vi "系统设置.vi"() -> ()   [LabVIEW 2016]
uses:
  <vilib>/Utility/miscctls.llb/LVPointTypeDef.ctl
  <vilib>/ptbypt/NI_PtbyPt.lvlib
  <vilib>/Utility/config.llb/NI_LVConfig.lvlib
  PLC/PLC.lvlib
  API/CodCr/CodCr.lvlib
panel:
  in  "质控周期":T1={"质控启动日期"="关闭", "跨度核查时间"=6, "空白核查时间"=2} {"跨度核查时间" items=["00H", "01H", "02H", "03H", "04H", "05H", "06H", "07H", "08H", "09H", "10H", "11H", "12H", "13H", "14H", "15H", "16H", "17H", "18H", "19H", "20H", "21H", "22H", "23H", "关闭"]; "空白核查时间" items=["00H", "01H", "02H", "03H", "04H", "05H", "06H", "07H", "08H", "09H", "10H", "11H", "12H", "13H", "14H", "15H", "16H", "17H", "18H", "19H", "20H", "21H", "22H", "23H", "关闭"]}
  in  "总氮启用":bool caption="总磷总氮禁用"
  in  "总氮":bool
  in  "超标留样启用":bool caption="质控单元禁用"
  in  "周期设置":enum16{"自由设定", "国标协议"}(ring)
  in  "运行间隔":i16=4 min=1 max=24
  out "x = y?":bool
  in  "CODCr":bool
  in  "总磷":bool
  in  "氨氮":bool
  in  "CODmn":bool
  in  "多参数":bool
  in  "24H周期设置":bool[](xcontrol)
  in  "输入密码":dbl
  in  "布尔":bool
  in  "副屏设置":bool
  in  "开机启动":bool caption="氨氮禁用"
  in  "CODMn启用":bool caption="CODMn禁用"
  in  "质控单元启用":bool caption="质控单元禁用"
  in  "总磷启用":bool caption="总磷总氮禁用"
  in  "流量计启用":bool caption="流量计禁用"
  in  "氨氮启用":bool caption="氨氮禁用"
  in  "多参数启用":bool caption="多参数禁用"
  in  "CODcr启用":bool caption="CODcr禁用"
  in  "运行模式":enum16{"维护模式", "常规模式", "应急模式", "质控模式"}(ring)
  # "注：周期设置分为自由设定和国标协议两种。\n1：选择自由设定情况下：运行间隔将不可选用并变灰色，周期设置可自由手动勾选\n2：选择国标协议情况下：周期时间将由运行间隔选择的时间决定，下方周期设置被禁用并无法手动勾选。"
  # "自动运行启动参数"
  # "启动周期设置"
  # "质控频次："
  # "空白核查时间："
  # "跨度核查时间："
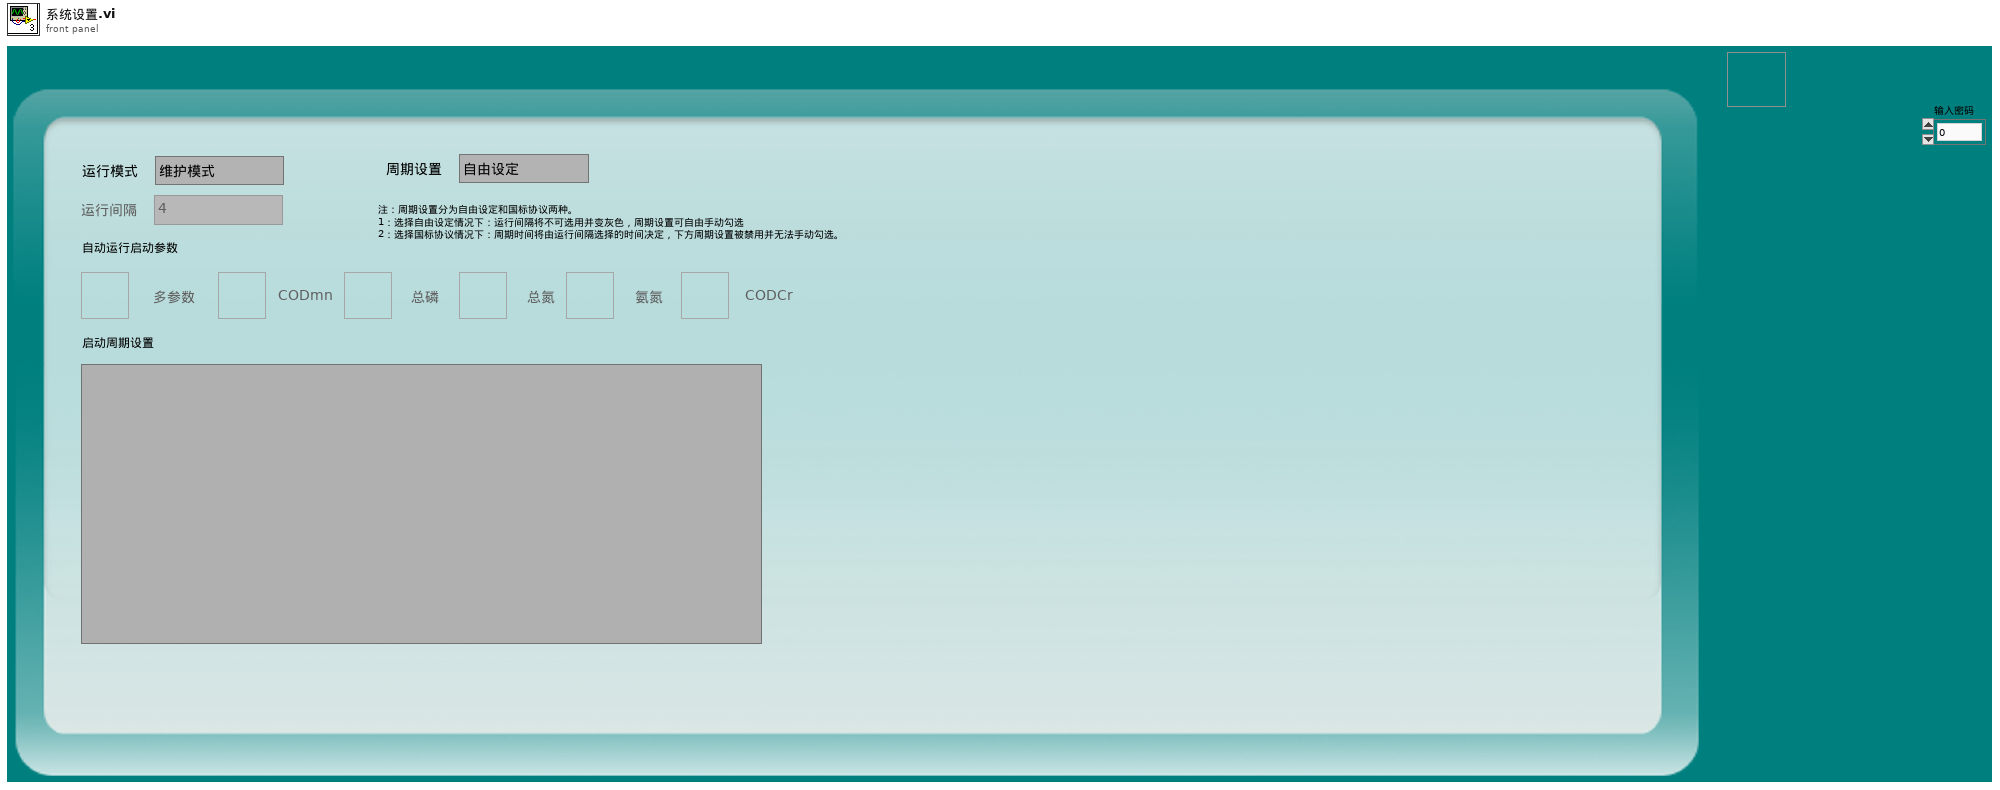
[diagram p1: front panel]
types:
  T1 = cluster{"质控启动日期":string, "跨度核查时间":u16, "空白核查时间":u16}
  T2 = typedef "LVPointTypeDef.ctl" = cluster{"Horizontal":i16, "Vertical":i16}
  T3 = typedef "NI_LVConfig.lvlib/Config Data RefNum.ctl" = refnum<k1>
  T4 = enum8{"Enabled", "Disabled", "Disabled and Grayed Out"}
  T5 = typedef "LVDateTimeRec.ctl" = cluster{"秒数的小数部分":dbl, "秒":i32, "分":i32, "时":i32, "日":i32, "月":i32, "年":i32, "天数（周）":i32, "天数（年）":i32, "DST":i32}
  T6 = enum32{"Invalid", "Standard", "Closed", "Hidden", "Minimized", "Maximized"}
  T7 = enum32{"Bad", "Idle", "Run top level", "Running"}
  T8 = cluster{"运行模式":enum16{"维护模式", "常规模式", "应急模式", "质控模式"}}
  T9 = cluster{"站号":u16, "量程切换":enum32{"H", "L", "AUTO"}, "控制命令":enum16{"启动测量", "标样核查", "零点核查", "跨度核查", "空白测试", "平行样测试", "加标回收", "空白校准", "标样校准", "初始化（清洗）", "停止测试", "仪器重启", "校时", "模式设置", "测量间隔设置"}, "模式设置":enum16{"待机", "连续模式", "周期模式", "定点模式", "受控模式", "手动模式"}, "测量间隔":u16}
  T10 = cluster{"测量模式":enum16{"水样测量", "标样核查", "零点核查", "跨度核查", "空白测试", "加标回收", "平行样", "校零", "校标"}}
  T11 = cluster{"水样测试量程切换模式":enum16{"H", "L", "AUTO"}, "空白核查量程切换模式":enum16{"H", "L", "AUTO"}, "跨度核查量程切换模式":enum16{"H", "L", "AUTO"}}
  T12 = cluster{"CODCr":cluster{"启动测量模式":cluster{"测量模式":enum16{"水样测量", "标样核查", "零点核查", "跨度核查", "空白测试", "加标回收", "平行样", "校零", "校标"}}, "确定按钮":bool}, "参数启用":cluster{"多参数":bool, "CODMn":bool, "总磷":bool, "总氮":bool, "氨氮":bool, "CODcr":bool}}
  T13 = cluster{"水样测试量程模式":enum16{"H", "L", "AUTO"}, "空白核查量程模式":enum16{"H", "L", "AUTO"}, "跨度核查量程模式":enum16{"H", "L", "AUTO"}}
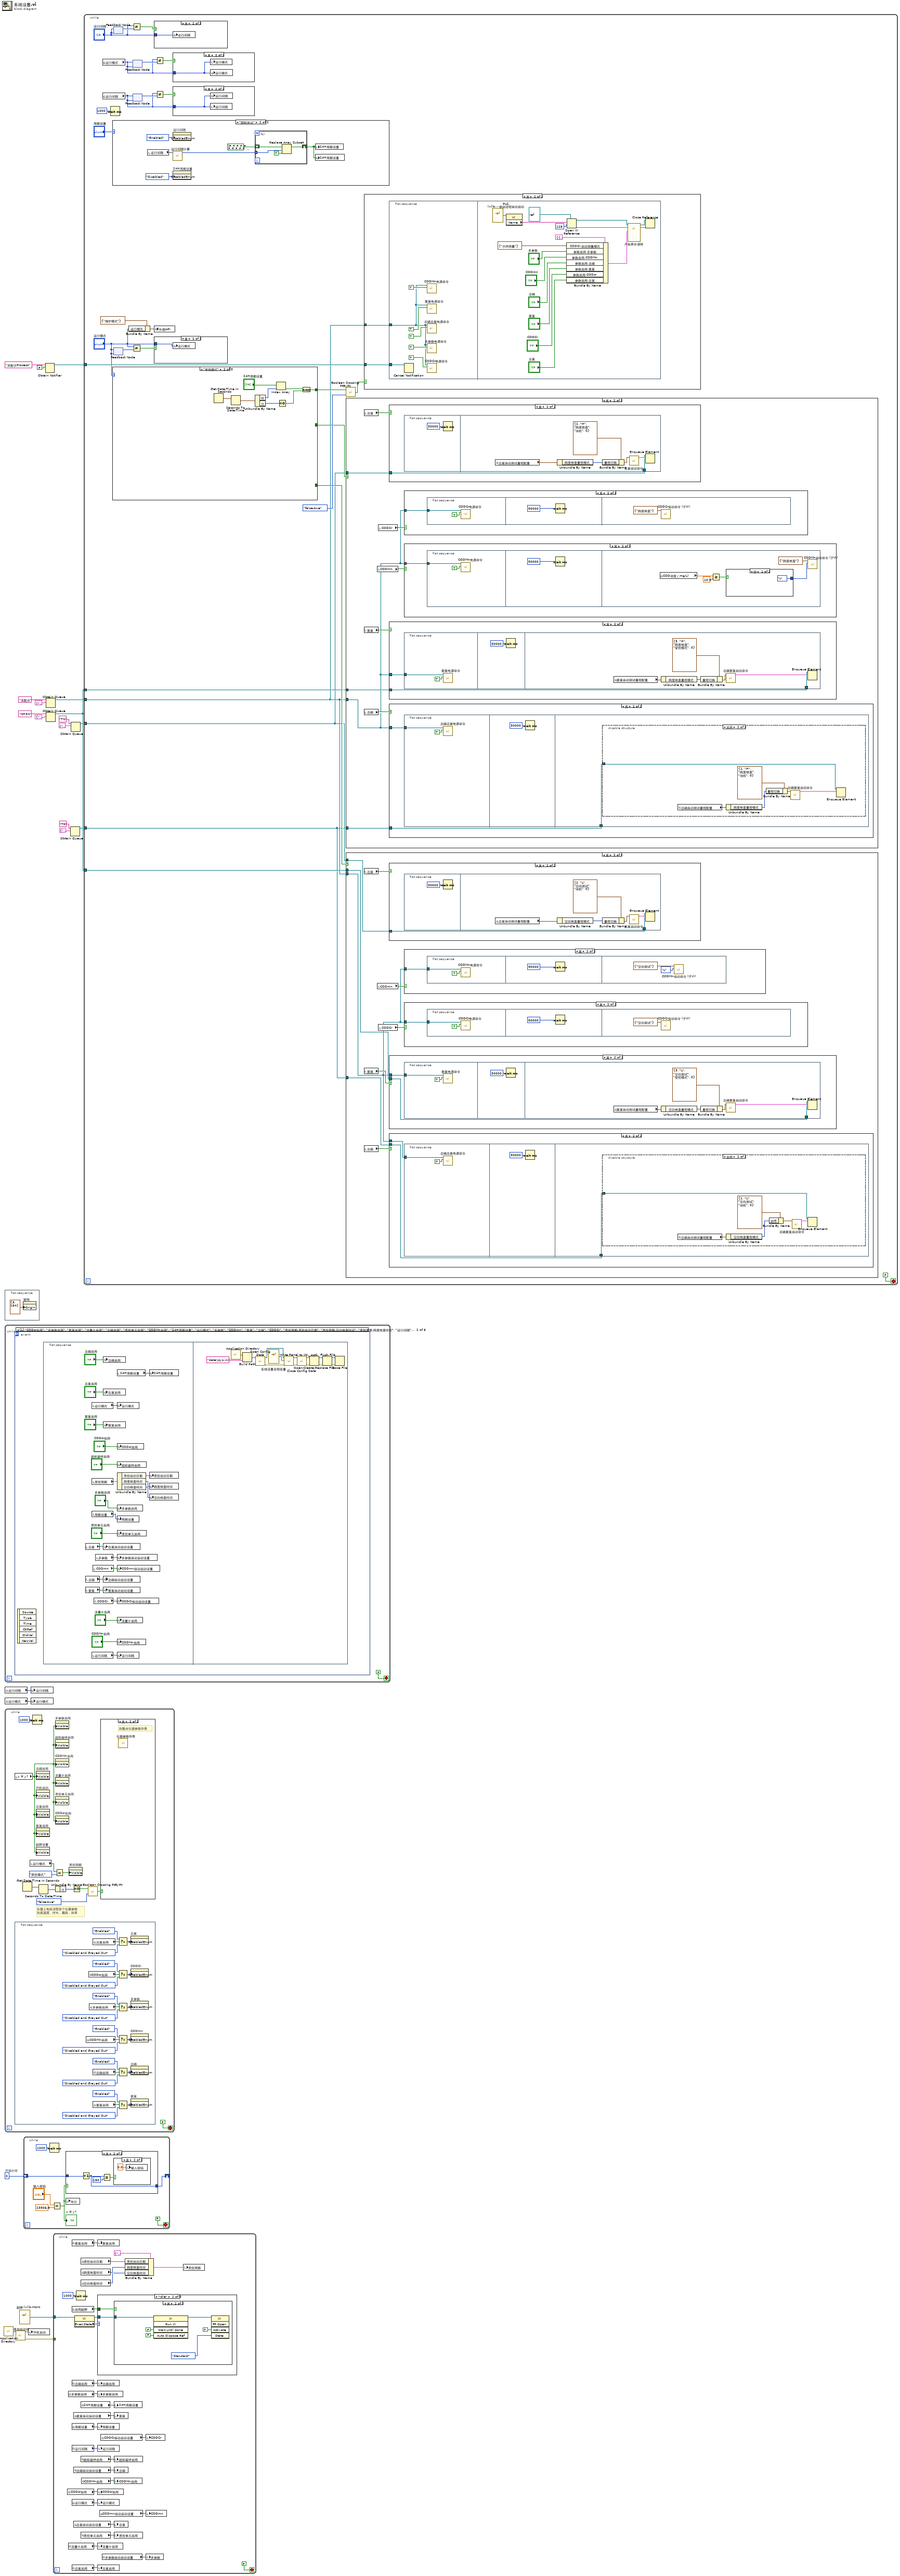
[diagram p0: block diagram]
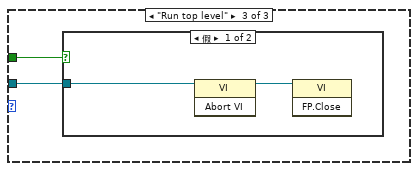
[diagram p7: hidden frame]
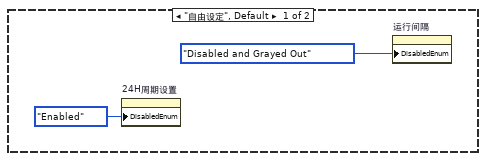
[diagram p9: hidden frame]
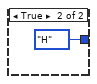
[diagram p18: hidden frame]
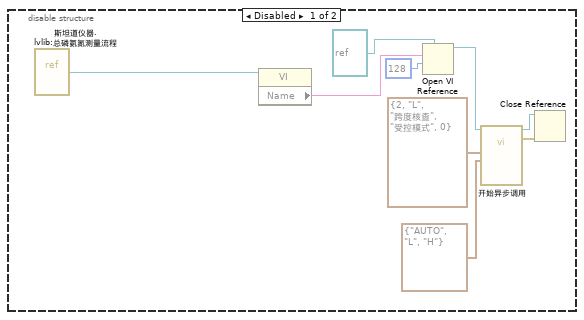
[diagram p20: hidden frame]
diagram:
  w16 = u32 0  # 开锁计时
  n1 = call <vilib>:"Application Directory.vi"() -> ("Application Directory"=w19:path)
  n2 = flat-sequence {
    frame #0 {
      n3 = property on="窗格" class="Pane"("Origin"=T2 {"Horizontal"=3, "Vertical"=164} ("原点")) -> ()  [unwired: 2 in, 2 out]
    }
  }
  n4 = while {
    stop <- FALSE stop-if-true
    n5 = event shown="[1] \"CODcr启用\", \"多参数启用\", \"氨氮启用\", \"流量计启用\", \"总磷启用\", \"质控单元启用\", \"CODMn启用\", \"24H周期设置\", \"运行模式\", \"多参数\", \"CODmn\", \"氨氮\", \"总磷\", \"CODCr\", \"质控周期.质控启动日期\", \"质控周期.空白核查时间\", \"质控周期.跨度核查时间\", \"运行间隔\", \"周期设置\", \"超标留样启用\", \"总氮\", \"总氮启用\": 值改变" {
      selector: _ -> [_ _ _ _ _ _]
      dyn-events: _ -> [_ _ _ _ _ _]
      timeout: _ -> [_ _ _ _ _ _]
      event Timeout {
        n6 = event-data() -> ()  [unwired: 1 in, 3 out]
      }
      event "CODcr启用", "多参数启用", "氨氮启用", "流量计启用", "总磷启用", "质控单元启用", "CODMn启用", "24H周期设置", "运行模式", "多参数", "CODmn", "氨氮", "总磷", "CODCr", "质控周期.质控启动日期", "质控周期.空白核查时间", "质控周期.跨度核查时间", "运行间隔", "周期设置", "超标留样启用", "总氮", "总氮启用": Value Change {
        n7 = event-data() -> ()  [unwired: 1 in, 6 out]
        n8 = flat-sequence {
          frame #0 {
            n9 = local read "总氮"() -> (w29:bool)
            n10 = local read "总磷"() -> (w37:bool)
            n11 = local read "氨氮"() -> (w39:bool)
            n12 = local read "运行模式"() -> (w40:enum16{"维护模式", "常规模式", "应急模式", "质控模式"})
            n13 = local read "质控周期"() -> (w28:T1)
            n14 = local read "周期设置"() -> (w32:enum16{"自由设定", "国标协议"})
            n15 = local read "运行间隔"() -> (w33:i16)
            n16 = local read "CODmn"() -> (w36:bool)
            n17 = local read "CODCr"() -> (w38:bool)
            n18 = local read "多参数"() -> (w35:bool)
            n19 = global write "系统设置全局变量.vi" "总磷启用"("总磷启用") -> ()
            n20 = global write "系统设置全局变量.vi" "总氮启用"("总氮启用") -> ()
            n21 = global write "系统设置全局变量.vi" "氨氮启用"("氨氮启用") -> ()
            n22 = global write "系统设置全局变量.vi" "总氮自动启动设置"(w29) -> ()
            n23 = global write "系统设置全局变量.vi" "总磷自动启动设置"(w37) -> ()
            n24 = global write "系统设置全局变量.vi" "氨氮自动启动设置"(w39) -> ()
            n25 = local read "24H周期设置"() -> (w34:bool[])
            n26 = global write "系统设置全局变量.vi" "运行模式"(w40) -> ()
            n27 = global write "系统设置全局变量.vi" "CODcr启用"("CODcr启用") -> ()
            n28 = global write "系统设置全局变量.vi" "超标留样启用"("超标留样启用") -> ()
            n29 = Unbundle By Name(w28) -> ("质控启动日期"=w27:string, "跨度核查时间"=w26:u16, "空白核查时间"=w25:u16)
            n30 = global write "系统设置全局变量.vi" "多参数启用"("多参数启用") -> ()
            n31 = global write "系统设置全局变量.vi" "周期设置"(w32) -> ()
            n32 = global write "系统设置全局变量.vi" "质控单元启用"("质控单元启用") -> ()
            n33 = global write "系统设置全局变量.vi" "多参数自动启动设置"(w35) -> ()
            n34 = global write "系统设置全局变量.vi" "CODmn自动启动设置"(w36) -> ()
            n35 = global write "系统设置全局变量.vi" "CODCr自动启动设置"(w38) -> ()
            n36 = global write "系统设置全局变量.vi" "流量计启用"("流量计启用") -> ()
            n37 = global write "系统设置全局变量.vi" "CODMn启用"("CODMn启用") -> ()
            n38 = global write "系统设置全局变量.vi" "运行间隔"(w33) -> ()
            n39 = global write "系统设置全局变量.vi" "24H周期设置"(w34) -> ()
            n40 = global write "系统设置全局变量.vi" "质控启动日期"(w27) -> ()
            n41 = global write "系统设置全局变量.vi" "跨度核查时间"(w26) -> ()
            n42 = global write "系统设置全局变量.vi" "空白核查时间"(w25) -> ()
          }
          frame #1 {
            n43 = call <vilib>:"Application Directory.vi"() -> ("Application Directory"=w61:path)
            n44 = Build Path(base path=w61, name or relative path="data\\sys.ini" ("名称或相对路径")) -> (appended path=w59:path)
            n45 = call <vilib>:"Open Config Data.vi"("configuration file path"=w59) -> ("error out"=w55:errorcluster, "refnum"=w58:T3)  [unwired: 8 in, 1 out]
            n46 = vi-ref "系统设置全局变量.vi"() -> (w57:refnum<vi>)
            n47 = call <userlib>:"Write Panel to INI__ogtk.vi"("error in (no error)"=w55, "VI ref"=w57, "refnum"=w58) -> ("error out"=w54:errorcluster, "refnum out"=w56:T3)  [unwired: 7 in]
            n48 = call <vilib>:"Close Config Data.vi"("error in (no error)"=w54, "refnum"=w56) -> ("error out"=w49:errorcluster, "file path"=w48:path)  [unwired: 8 in]
            n49 = Open/Create/Replace File(file path (use dialog)=w48, error in=w49) -> (refnum out=w52:refnum<file>, error out=w53:errorcluster)  [unwired: 4 in, 1 out]
            n50 = Flush File(refnum=w52, error in=w53) -> (refnum out=w51:refnum<file>, error out=w50:errorcluster)
            n51 = Close File(refnum=w51, error in=w50) -> ()  [unwired: 2 out]
          }
        }
      }
      event "运行间隔": Mouse Down {
        n52 = event-data() -> ("CtlRef"=w65:refnum<vi>)  [unwired: 1 in, 7 out]
        n53 = property class="DigNum (严格)"(reference=w65) -> (reference out=w64:refnum<vi>, "Value"=w63:i16)  [unwired: 1 in, 1 out]
        n54 = call "数字键盘.vi"("OldNumber"=w63) -> ("NewNumber"=w62:sgl)
        n55 = property class="DigNum (严格)"(reference=w64, "Val(Sgnl)"=w62) -> ()  [unwired: 1 in, 2 out]
      }
      event "开机启动": Value Change {
        n56 = event-data() -> ("NewVal"=w67:bool)  [unwired: 1 in, 5 out]
        n57 = call <vilib>:"Application Directory.vi"() -> ("Application Directory"=w66:path)
        n58 = case shown="假" w67 {
          tunnel: w66 -> [w69 w73]
          frame False {
            n59 = call "删除启动项.vi"("启动文件路径"=w69) -> ("删除标记"=w68:bool)  [unwired: 9 in, 1 out]
            n60 = case shown="假" w68 {
              frame False {
                n61 = local write "开机启动"(TRUE ("开机启动")) -> ()
                n62 = One Button Dialog(message="启动项删除失败" ("消息")) -> ()  [unwired: 1 in, 1 out]
              }
              frame True {
              }
            }
          }
          frame True {
            n63 = call "添加启动项.vi"("启动文件路径"=w73) -> ("添加成功标记"=w72:bool)  [unwired: 9 in, 1 out]
            n64 = case shown="假" w72 {
              frame False {
                n65 = local write "开机启动"(FALSE ("开机启动")) -> ()
                n66 = One Button Dialog(message="启动项添加失败" ("消息")) -> ()  [unwired: 1 in, 1 out]
              }
              frame True {
              }
            }
          }
        }
      }
      event "副屏设置": Value Change {
        n67 = event-data() -> ()  [unwired: 1 in, 6 out]
        n68 = call "副屏设置.vi"() -> ()  [unwired: 12 in]
      }
      event "布尔": Value Change {
        n69 = event-data() -> ("OldVal"=w77:bool)  [unwired: 1 in, 5 out]
        n70 = case shown="假" w77 {
          tunnel: [w78 _] -> w76
          frame False {
            n71 = call "数字密码键盘.vi"() -> ("NewNumber"=w78:sgl)  [unwired: 1 in]
          }
          frame True {
          }
        }
        n72 = local write "输入密码"(w76) -> ()
      }
    }
  }
  n73 = global read "系统设置全局变量.vi" "运行间隔"() -> (w2:i16)
  n74 = global read "系统设置全局变量.vi" "运行模式"() -> (w1:enum16{"维护模式", "常规模式", "应急模式", "质控模式"})
  n75 = while {
    stop <- FALSE stop-if-true
    # "仪器上电就读取各个仪器参数\n包括温度，时长，截距，斜率"
    n76 = local read "x = y?"() -> (w82:bool)
    n77 = flat-sequence {
      frame #0 {
        n78 = global read "系统设置全局变量.vi" "CODMn启用"() -> (w99:bool)
        n79 = global read "系统设置全局变量.vi" "CODcr启用"() -> (w100:bool)
        n80 = global read "系统设置全局变量.vi" "多参数启用"() -> (w98:bool)
        n81 = global read "系统设置全局变量.vi" "总氮启用"() -> (w94:bool)
        n82 = global read "系统设置全局变量.vi" "总磷启用"() -> (w101:bool)
        n83 = global read "系统设置全局变量.vi" "氨氮启用"() -> (w97:bool)
        n84 = Select(t=T4."Enabled" ("禁用"), s=w94, f=T4."Disabled and Grayed Out" ("禁用")) -> (s? t:f=w91:T4)
        n85 = Select(t=T4."Enabled" ("禁用"), s=w100, f=T4."Disabled and Grayed Out" ("禁用")) -> (s? t:f=w114:T4)
        n86 = Select(t=T4."Enabled" ("禁用"), s=w98, f=T4."Disabled and Grayed Out" ("禁用")) -> (s? t:f=w96:T4)
        n87 = Select(t=T4."Enabled" ("禁用"), s=w99, f=T4."Disabled and Grayed Out" ("禁用")) -> (s? t:f=w103:T4)
        n88 = Select(t=T4."Enabled" ("禁用"), s=w101, f=T4."Disabled and Grayed Out" ("禁用")) -> (s? t:f=w95:T4)
        n89 = Select(t=T4."Enabled" ("禁用"), s=w97, f=T4."Disabled and Grayed Out" ("禁用")) -> (s? t:f=w102:T4)
        n90 = property on="总氮" class="Bool (严格)"("DisabledEnum"=w91) -> ()  [unwired: 2 in, 2 out]
        n91 = property on="CODCr" class="Bool (严格)"("DisabledEnum"=w114) -> ()  [unwired: 2 in, 2 out]
        n92 = property on="多参数" class="Bool (严格)"("DisabledEnum"=w96) -> ()  [unwired: 2 in, 2 out]
        n93 = property on="CODmn" class="Bool (严格)"("DisabledEnum"=w103) -> ()  [unwired: 2 in, 2 out]
        n94 = property on="总磷" class="Bool (严格)"("DisabledEnum"=w95) -> ()  [unwired: 2 in, 2 out]
        n95 = property on="氨氮" class="Bool (严格)"("DisabledEnum"=w102) -> ()  [unwired: 2 in, 2 out]
      }
    }
    n96 = Get Date/Time In Seconds() -> (seconds since 1Jan1904=w88:timestamp)
    n97 = local read "运行模式"() -> (w81:enum16{"维护模式", "常规模式", "应急模式", "质控模式"})
    n98 = Wait (ms)(milliseconds to wait=u32 1000 ("等待时间（毫秒）")) -> ()  [unwired: 1 out]
    n99 = property on="总磷启用" class="Bool (严格)"("Visible"=w82) -> ()  [unwired: 2 in, 2 out]
    n100 = property on="开机启动" class="Bool (严格)"("Visible"=w82) -> ()  [unwired: 2 in, 2 out]
    n101 = property on="总氮启用" class="Bool (严格)"("Visible"=w82) -> ()  [unwired: 2 in, 2 out]
    n102 = property on="氨氮启用" class="Bool (严格)"("Visible"=w82) -> ()  [unwired: 2 in, 2 out]
    n103 = property on="副屏设置" class="Bool"("Visible"=w82) -> ()  [unwired: 2 in, 2 out]
    n104 = Seconds To Date/Time(time stamp (now)=w88) -> (date time rec=w87:T5)  [unwired: 1 in]
    n105 = Equal?(x=w81, y=enum16{"维护模式", "常规模式", "应急模式", "质控模式"}."质控模式") -> (x = y?=w79:bool)
    n106 = property on="多参数启用" class="Bool (严格)"("Visible"=w82) -> ()  [unwired: 2 in, 2 out]
    n107 = property on="超标留样启用" class="Bool (严格)"("Visible"=w82) -> ()  [unwired: 2 in, 2 out]
    n108 = property on="CODMn启用" class="Bool (严格)"("Visible"=w82) -> ()  [unwired: 2 in, 2 out]
    n109 = property on="流量计启用" class="Bool (严格)"("Visible"=w82) -> ()  [unwired: 2 in, 2 out]
    n110 = property on="质控单元启用" class="Bool (严格)"("Visible"=w82) -> ()  [unwired: 2 in, 2 out]
    n111 = property on="CODcr启用" class="Bool (严格)"("Visible"=w82) -> ()  [unwired: 2 in, 2 out]
    n112 = Unbundle By Name(w87) -> ("分"=w86:i32)
    n113 = property on="质控周期" class="Clust (严格)"("Visible"=w79) -> ()  [unwired: 2 in, 2 out]
    n114 = Equal To 0?(x=w86) -> (x = 0?=w85:bool)
    n115 = call <vilib>:"Boolean Crossing PtByPt.vi"("direction"=enum16{"either", "false-true", "true-false"}."false-true", "input"=w85) -> ("crossing"=w83:bool)  [unwired: 1 in]
    n116 = case shown="真" w83 {
      frame False {
      }
      frame True {
        # "到整点仪器参数存表"
        n117 = call "仪器参数存表.vi"() -> ()  [unwired: 12 in]
      }
    }
  }
  n118 = call "查询启动项.vi"("启动文件路径"=w19) -> ("error out"=w17:errorcluster, "包含启动项"=w18:bool)  [unwired: 9 in]
  n119 = vi-ref "副屏.lvlib:MAIN.vi"() -> (w12:refnum<vi>)
  n120 = while {
    shift-right: [w116] -> _
    shift-left: w16 -> [w117]
    stop <- FALSE stop-if-true
    n121 = Wait (ms)(milliseconds to wait=u32 1000 ("等待时间（毫秒）")) -> ()  [unwired: 1 out]
    n122 = Equal?(x="输入密码", y=23506.0) -> (x = y?=w115:bool)
    "x = y?" <- w115
    n123 = case shown="真" w115 {
      tunnel: w117 -> [_ w125]
      tunnel: [_ w124] -> w116
      frame False {
      }
      frame True {
        n124 = Increment(x=w125) -> (x+1=w124:u32)
        n125 = Greater Or Equal?(x=w124, y=u32 180) -> (x >= y?=w122:bool)
        n126 = case shown="真" w122 {
          frame False {
          }
          frame True {
            n127 = local write "输入密码"(0.0 ("输入密码")) -> ()
          }
        }
      }
    }
    n128 = local write "布尔"(w115) -> ()
  }
  n129 = local write "开机启动"(w18) -> ()
  n130 = global write "系统变量.vi" "运行间隔"(w2) -> ()
  n131 = global write "系统变量.vi" "运行模式"(w1) -> ()
  n132 = Obtain Notifier(name (unnamed)="采配水Process" ("名称（未命名）"), notification data type=FALSE) -> (notifier out=w20:refnum<notifier>)  [unwired: 2 in, 2 out]
  n133 = Obtain Queue(name (unnamed)="采配水" ("名称（未命名）"), element data type=cluster{"命令":string, "数据":variant} {"命令"="", "数据"=variant}) -> (queue out=w13:refnum<queue>)  [unwired: 3 in, 2 out]
  n134 = Obtain Queue(name (unnamed)="NH3N" ("名称（未命名）"), element data type=cluster{"命令":string, "data":variant} {"命令"="", "data"=variant}) -> (queue out=w9:refnum<queue>)  [unwired: 3 in, 2 out]
  n135 = while {
    tunnel: w17 -> [_]
    tunnel: w12 -> [w140]
    stop <- FALSE stop-if-true
    n136 = global read "系统设置全局变量.vi" "CODcr启用"() -> (w149:bool)
    n137 = global read "系统设置全局变量.vi" "多参数启用"() -> (w148:bool)
    n138 = global read "系统设置全局变量.vi" "流量计启用"() -> (w150:bool)
    n139 = global read "系统设置全局变量.vi" "氨氮启用"() -> (w154:bool)
    n140 = global read "副屏设置全局变量.vi" "启用副屏"() -> (w138:bool)
    n141 = global read "系统设置全局变量.vi" "总磷启用"() -> (w151:bool)
    n142 = global read "系统设置全局变量.vi" "周期设置"() -> (w135:enum16{"自由设定", "国标协议", "流量设定"})
    n143 = global read "系统设置全局变量.vi" "运行间隔"() -> (w136:i16)
    n144 = global read "系统设置全局变量.vi" "运行模式"() -> (w146:enum16{"维护模式", "常规模式", "应急模式", "质控模式"})
    n145 = global read "系统设置全局变量.vi" "总氮启用"() -> (w133:bool)
    n146 = global read "系统设置全局变量.vi" "氨氮自动启动设置"() -> (w145:bool)
    n147 = global read "系统设置全局变量.vi" "总磷自动启动设置"() -> (w143:bool)
    n148 = global read "系统设置全局变量.vi" "总氮自动启动设置"() -> (w132:bool)
    n149 = property class="VI"(reference=w140) -> (reference out=w137:refnum<vi>, "Exec.State"=w139:T7)  [unwired: 1 in, 1 out]
    n150 = Wait (ms)(milliseconds to wait=u32 1000 ("等待时间（毫秒）")) -> ()  [unwired: 1 out]
    n151 = global read "系统设置全局变量.vi" "质控启动日期"() -> (w129:string)
    n152 = global read "系统设置全局变量.vi" "跨度核查时间"() -> (w128:u16)
    n153 = global read "系统设置全局变量.vi" "空白核查时间"() -> (w127:u16)
    n154 = global read "系统设置全局变量.vi" "24H周期设置"() -> (w147:bool[])
    n155 = global read "系统设置全局变量.vi" "超标留样启用"() -> (w134:bool)
    n156 = global read "系统设置全局变量.vi" "质控单元启用"() -> (w152:bool)
    n157 = global read "系统设置全局变量.vi" "CODMn启用"() -> (w153:bool)
    n158 = local write "氨氮启用"(w154) -> ()
    n159 = case shown="\"Idle\"" w139 {
      tunnel: w138 -> [_ w157 w165]
      tunnel: w137 -> [_ w158 w166]
      frame "Bad", Default {
      }
      frame "Idle" {
        n160 = case shown="真" w157 {
          tunnel: w158 -> [_ w164]
          frame False {
          }
          frame True {
            n161 = invoke class="VI" method="Run VI"(reference=w164, "Wait until done"=FALSE ("结束前等待"), "Auto Dispose Ref"=FALSE ("自动销毁引用")) -> (reference out=w159:refnum<vi>)  [unwired: 2 in, 4 out]
            n162 = invoke class="VI" method="FP.Open"(reference=w159, "Activate"=TRUE ("激活？"), "State"=T6."Standard" ("状态")) -> ()  [unwired: 2 in, 5 out]
          }
        }
      }
      frame "Run top level" {
        n163 = case shown="假" w165 {
          tunnel: w166 -> [w167 _]
          frame False {
            n164 = invoke class="VI" method="Abort VI"(reference=w167) -> (reference out=w168:refnum<vi>)  [unwired: 2 in, 2 out]
            n165 = invoke class="VI" method="FP.Close"(reference=w168) -> ()  [unwired: 2 in, 3 out]
          }
          frame True {
          }
        }
      }
    }
    n166 = local write "总磷启用"(w151) -> ()
    n167 = local write "多参数启用"(w148) -> ()
    n168 = local write "周期设置"(w135) -> ()
    n169 = local write "运行间隔"(w136) -> ()
    n170 = local write "CODcr启用"(w149) -> ()
    n171 = local write "运行模式"(w146) -> ()
    n172 = local write "流量计启用"(w150) -> ()
    n173 = local write "总氮启用"(w133) -> ()
    n174 = global read "系统设置全局变量.vi" "CODmn自动启动设置"() -> (w142:bool)
    n175 = global read "系统设置全局变量.vi" "CODCr自动启动设置"() -> (w144:bool)
    n176 = global read "系统设置全局变量.vi" "多参数自动启动设置"() -> (w141:bool)
    n177 = local write "24H周期设置"(w147) -> ()
    n178 = local write "氨氮"(w145) -> ()
    n179 = local write "超标留样启用"(w134) -> ()
    n180 = local write "总磷"(w143) -> ()
    n181 = local write "CODMn启用"(w153) -> ()
    n182 = local write "总氮"(w132) -> ()
    n183 = local write "质控单元启用"(w152) -> ()
    n184 = Bundle By Name(cluster=T1 {"质控启动日期"="关闭", "跨度核查时间"=24, "空白核查时间"=24} ("质控周期"), "质控启动日期"=w129, "跨度核查时间"=w128, "空白核查时间"=w127) -> (w130:T1)
    n185 = local write "CODCr"(w144) -> ()
    n186 = local write "CODmn"(w142) -> ()
    n187 = local write "多参数"(w141) -> ()
    n188 = local write "质控周期"(w130) -> ()
  }
  n189 = Obtain Queue(name (unnamed)="TP" ("名称（未命名）"), element data type=cluster{"命令":string, "data":variant} {"命令"="", "data"=variant}) -> (queue out=w4:refnum<queue>)  [unwired: 3 in, 2 out]
  n190 = Obtain Queue(name (unnamed)="TN" ("名称（未命名）"), element data type=cluster{"命令":string, "data":variant} {"命令"="", "data"=variant}) -> (queue out=w3:refnum<queue>)  [unwired: 3 in, 2 out]
  n191 = while {
    tunnel: w20 -> [w194]
    tunnel: w13 -> [w186]
    tunnel: w9 -> [w185]
    tunnel: w9 -> [w184]
    tunnel: w4 -> [w170]
    tunnel: w3 -> [w169]
    stop <- FALSE stop-if-true
    n192 = global read "系统变量.vi" "运行模式"() -> (w178:enum16{"维护模式", "常规模式", "应急模式", "质控模式"})
    n193 = global read "系统变量.vi" "运行间隔"() -> (w172:i16)
    n194 = Wait (ms)(milliseconds to wait=u32 1000 ("等待时间（毫秒）")) -> ()  [unwired: 1 out]
    n195 = case shown="\"国标协议\"" "周期设置" {
      frame "自由设定", Default {
        n196 = property on="24H周期设置" class="24H周期设置 (严格)"("DisabledEnum"=T4."Enabled" ("禁用")) -> ()  [unwired: 2 in, 2 out]
        n197 = property on="运行间隔" class="DigNum (严格)"("DisabledEnum"=T4."Disabled and Grayed Out" ("禁用")) -> ()  [unwired: 2 in, 2 out]
      }
      frame "国标协议" {
        n198 = local read "运行间隔"() -> (w204:i16)
        n199 = property on="运行间隔" class="DigNum (严格)"("DisabledEnum"=T4."Enabled" ("禁用")) -> ()  [unwired: 2 in, 2 out]
        n200 = call "运行间隔计算.vi"("运行周期"=w204) -> ("数组"=w203:i32[])  [unwired: 10 in]
        n201 = property on="24H周期设置" class="24H周期设置 (严格)"("DisabledEnum"=T4."Disabled" ("禁用")) -> ()  [unwired: 2 in, 2 out]
        n202 = for {
          tunnel: w203 -> [w207] mode=indexing
          shift-right: [w205] -> w201
          shift-left: bool[] [FALSE, FALSE, FALSE, FALSE, FALSE, FALSE, FALSE, FALSE, FALSE, FALSE, FALSE, FALSE, FALSE, FALSE, FALSE, FALSE, FALSE, FALSE, FALSE, FALSE, FALSE, FALSE, FALSE, FALSE] ("24H周期设置") -> [w208]
          n203 = Replace Array Subset(array=w208, new element=TRUE ("新元素/子数组"), index=w207) -> (w205:bool[])
        }
        n204 = local write "24H周期设置"(w201) -> ()
        n205 = global write "系统设置全局变量.vi" "24H周期设置"(w201) -> ()
      }
    }
    n206 = case shown="\"常规模式\"" "运行模式" {
      tunnel: [_ w367 w378] -> w193
      tunnel: [_ _ w377] -> w187
      tunnel: [_ _ w376] -> w188
      frame "维护模式", Default {
      }
      frame "常规模式" {
        n207 = Get Date/Time In Seconds() -> (seconds since 1Jan1904=w371:timestamp)
        n208 = Seconds To Date/Time(time stamp (now)=w371) -> (date time rec=w370:T5)  [unwired: 1 in]
        n209 = Unbundle By Name(w370) -> ("时"=w365:i32, "分"=w369:i32)
        n210 = Index Array(array="24H周期设置", index=w365) -> (element=w364:bool)
        n211 = Equal To 0?(x=w369) -> (x = 0?=w368:bool)
        n212 = And(x=w364, y=w368) -> (x .and. y?=w367:bool)
      }
      frame "质控模式" {
        # "跨度"
        # "零点"
        n213 = Get Date/Time In Seconds() -> (seconds since 1Jan1904=w386:timestamp)
        n214 = Format Date/Time String(time format string (%c)="%A" ("时间格式字符串(%c)"), seconds (now)=w386) -> (date/time string=w384:string)  [unwired: 1 in]
        n215 = Unbundle By Name("质控周期") -> ("质控启动日期"=w375:string, "跨度核查时间"=w372:u16, "空白核查时间"=w373:u16)
        n216 = case shown="\"每天\"" w375 {
          selector: w375 -> [w401 _ _]
          tunnel: [w400 TRUE FALSE] -> w387
          tunnel: w384 -> [w399 _ _]
          frame "星期二", "星期六", "星期日", "星期三", "星期四", "星期五", "星期一" {
            n217 = Equal?(x=w399, y=w401) -> (x = y?=w400:bool)
          }
          frame "每天" {
          }
          frame "关闭", Default {
          }
        }
        n218 = Seconds To Date/Time(time stamp (now)=w386) -> (date time rec=w398:T5)  [unwired: 1 in]
        n219 = local read "24H周期设置"() -> (w381:bool[])
        n220 = Unbundle By Name(w398) -> ("时"=w379:i32, "分"=w397:i32, "时"=w395:i32, "分"=w394:i32, "时"=w391:i32, "分"=w390:i32, "秒"=w383:i32)
        n221 = Equal?(x=w391, y=w372) -> (x = y?=w389:bool)
        n222 = Equal?(x=w395, y=w373) -> (x = y?=w393:bool)
        n223 = Index Array(array=w381, index=w379) -> (element=w380:bool)
        n224 = Equal To 0?(x=w397) -> (x = 0?=w396:bool)
        n225 = And(x=w380, y=w396) -> (x .and. y?=w378:bool)
        n226 = Equal To 0?(x=w390) -> (x = 0?=w388:bool)
        n227 = Equal To 0?(x=w394) -> (x = 0?=w392:bool)
        n228 = Equal To 0?(x=w383) -> (x = 0?=w382:bool)
        n229 = Compound Arithmetic op=AND ("复合运算")(w389, w388, w387, w382) -> (w377:bool)
        n230 = Compound Arithmetic op=AND ("复合运算")(w392, w393, w387, w382) -> (w376:bool)
      }
    }
    n231 = feedback #1("运行间隔") -> (w177:i16)
    n232 = feedback-in #1("运行间隔") -> ()
    n233 = feedback-in #2("运行模式") -> ()
    n234 = feedback #2("运行模式") -> (w183:enum16{"维护模式", "常规模式", "应急模式", "质控模式"})
    n235 = Bundle By Name(cluster=T8 {"运行模式"=enum."维护模式"} ("外围API"), "运行模式"="运行模式") -> (w189:T8)
    n236 = Not Equal?(x="运行间隔", y=w177) -> (x != y?=w176:bool)
    n237 = Not Equal?(x="运行模式", y=w183) -> (x != y?=w182:bool)
    n238 = feedback #3(w178) -> (w180:enum16{"维护模式", "常规模式", "应急模式", "质控模式"})
    n239 = feedback-in #3(w178) -> ()
    n240 = feedback #4(w172) -> (w174:i16)
    n241 = feedback-in #4(w172) -> ()
    n242 = case shown="真" w176 {
      tunnel: "运行间隔" -> [_ w210]
      frame False {
      }
      frame True {
        n243 = global write "系统变量.vi" "运行间隔"(w210) -> ()
      }
    }
    n244 = global write "VAR总磷氨氮全局变量.vi" "外围API"(w189) -> ()
    n245 = case shown="真" w182 {
      tunnel: "运行模式" -> [_ w212]
      frame False {
      }
      frame True {
        n246 = global write "系统变量.vi" "运行模式"(w212) -> ()
      }
    }
    n247 = Not Equal?(x=w178, y=w180) -> (x != y?=w179:bool)
    n248 = Not Equal?(x=w172, y=w174) -> (x != y?=w173:bool)
    n249 = case shown="真" w179 {
      tunnel: w178 -> [_ w211]
      frame False {
      }
      frame True {
        n250 = local write "运行模式"(w211) -> ()
        n251 = global write "系统设置全局变量.vi" "运行模式"(w211) -> ()
      }
    }
    n252 = case shown="真" w173 {
      tunnel: w172 -> [_ w209]
      frame False {
      }
      frame True {
        n253 = global write "系统设置全局变量.vi" "运行间隔"(w209) -> ()
        n254 = local write "运行间隔"(w209) -> ()
      }
    }
    n255 = call <vilib>:"Boolean Crossing PtByPt.vi"("direction"=enum16{"either", "false-true", "true-false"}."false-true", "input"=w193) -> ("crossing"=w191:bool)  [unwired: 1 in]
    n256 = case shown="真" w187 {
      tunnel: w186 -> [_ w217]
      tunnel: w184 -> [_ w216]
      tunnel: w170 -> [_ w215]
      tunnel: w169 -> [_ w213]
      frame False {
      }
      frame True {
        n257 = local read "总氮"() -> (w214:bool)
        n258 = local read "氨氮"() -> (w221:bool)
        n259 = local read "总磷"() -> (w220:bool)
        n260 = local read "CODmn"() -> (w219:bool)
        n261 = local read "CODCr"() -> (w218:bool)
        n262 = case shown="真" w214 {
          tunnel: w213 -> [_ w222]
          frame False {
          }
          frame True {
            n263 = flat-sequence {
              tunnel: w222 -> [w228]
              frame #0 {
                n264 = Wait (ms)(milliseconds to wait=u32 30000 ("等待时间（毫秒）")) -> ()  [unwired: 1 out]
              }
              frame #1 {
                n265 = global read "系统设置全局变量.vi" "总氮自动测试量程配置"() -> (w225:T13)
                n266 = Unbundle By Name(w225) -> ("跨度核查量程模式"=w224:enum16{"H", "L", "AUTO"})
                n267 = Bundle By Name(cluster=T9 {"站号"=2, "量程切换"=enum."H", "控制命令"=enum."跨度核查", "模式设置"=enum."待机", "测量间隔"=0} ("参数"), "量程切换"=w224) -> (w226:T9)
                n268 = call "总氮启动命令.vi"("参数"=w226) -> ("启动命令"=w229:cluster{"命令":string, "data":variant})  [unwired: 10 in]
                n269 = Enqueue Element(queue=w228, element=w229) -> ()  [unwired: 2 in, 3 out]
              }
            }
          }
        }
        n270 = case shown="真" w221 {
          tunnel: w217 -> [_ w268]
          tunnel: w216 -> [_ w267]
          frame False {
          }
          frame True {
            n271 = flat-sequence {
              tunnel: w268 -> [w269]
              tunnel: w267 -> [w276]
              frame #0 {
                n272 = call "氨氮电源命令.vi"("通电/断电"=TRUE, "队列"=w269) -> ()  [unwired: 9 in, 1 out]
              }
              frame #1 {
                n273 = Wait (ms)(milliseconds to wait=u32 30000 ("等待时间（毫秒）")) -> ()  [unwired: 1 out]
              }
              frame #2 {
                n274 = global read "系统设置全局变量.vi" "氨氮自动测试量程配置"() -> (w273:T13)
                n275 = Unbundle By Name(w273) -> ("跨度核查量程模式"=w272:enum16{"H", "L", "AUTO"})
                n276 = Bundle By Name(cluster=T9 {"站号"=3, "量程切换"=enum."H", "控制命令"=enum."跨度核查", "模式设置"=enum."受控模式", "测量间隔"=0} ("参数"), "量程切换"=w272) -> (w274:T9)
                n277 = call "总磷氨氮启动命令.vi"("参数"=w274) -> ("启动命令"=w277:cluster{"命令":string, "data":variant})  [unwired: 10 in]
                n278 = Enqueue Element(queue=w276, element=w277) -> ()  [unwired: 2 in, 3 out]
              }
            }
          }
        }
        n279 = case shown="真" w220 {
          tunnel: w217 -> [_ w247]
          tunnel: w215 -> [_ w246]
          frame False {
          }
          frame True {
            n280 = flat-sequence {
              tunnel: w247 -> [w249]
              tunnel: w246 -> [w251]
              frame #0 {
                n281 = call "总磷总氮电源命令.vi"("通电/断电"=TRUE, "队列"=w249) -> ()  [unwired: 9 in, 1 out]
              }
              frame #1 {
                n282 = Wait (ms)(milliseconds to wait=u32 30000 ("等待时间（毫秒）")) -> ()  [unwired: 1 out]
              }
              frame #2 {
                n283 = disable-structure shown="启用" {
                  disable-tunnel: w251 -> [_ w265]
                  frame Disabled {
                    n284 = vi-ref "斯坦道仪器.lvlib:总磷氨氮测量流程.vi"() -> (w257:refnum<vi>)
                    n285 = property class="VI"(reference=w257) -> ("Name"=w258:string)  [unwired: 1 in, 2 out]
                    n286 = Open VI Reference(type specifier VI Refnum (for type only)=refnum<vi> refnum ("类型说明符VI引用句柄（仅用于类型）"), vi path=w258, options=128 ("选项")) -> (vi reference=w256:refnum<vi>)  [unwired: 3 in, 1 out]
                    n287 = call-by-ref "开始异步调用"(reference=w256, "量程模式"=T11 {"水样测试量程切换模式"=enum."AUTO", "空白核查量程切换模式"=enum."L", "跨度核查量程切换模式"=enum."H"}, "参数"=T9 {"站号"=2, "量程切换"=enum."L", "控制命令"=enum."跨度核查", "模式设置"=enum."受控模式", "测量间隔"=0}) -> (reference out=w253:refnum<vi>, error out=w252:errorcluster)  [unwired: 11 in]
                    n288 = Close Reference(reference=w253, error in (no error)=w252) -> ()  [unwired: 1 out]
                  }
                  frame Enabled {
                    n289 = global read "系统设置全局变量.vi" "总磷自动测试量程配置"() -> (w262:T13)
                    n290 = Unbundle By Name(w262) -> ("跨度核查量程模式"=w261:enum16{"H", "L", "AUTO"})
                    n291 = Bundle By Name(cluster=T9 {"站号"=1, "量程切换"=enum."H", "控制命令"=enum."跨度核查", "模式设置"=enum."待机", "测量间隔"=0} ("参数"), "量程切换"=w261) -> (w263:T9)
                    n292 = call "总磷氨氮启动命令.vi"("参数"=w263) -> ("启动命令"=w266:cluster{"命令":string, "data":variant})  [unwired: 10 in]
                    n293 = Enqueue Element(queue=w265, element=w266) -> ()  [unwired: 2 in, 3 out]
                  }
                }
              }
            }
          }
        }
        n294 = case shown="真" w218 {
          tunnel: w217 -> [_ w230]
          frame False {
          }
          frame True {
            n295 = flat-sequence {
              tunnel: w230 -> [w231]
              frame #0 {
                n296 = call "CODCr电源命令.vi"("通电/断电"=TRUE, "队列"=w231) -> ()  [unwired: 9 in, 1 out]
              }
              frame #1 {
                n297 = Wait (ms)(milliseconds to wait=u32 90000 ("等待时间（毫秒）")) -> ()  [unwired: 1 out]
              }
              frame #2 {
                n298 = call "CODCr启动命令 (子VI).vi"("启动测量模式"=T10 {"测量模式"=enum."跨度核查"}) -> ()  [unwired: 11 in]
              }
            }
          }
        }
        n299 = case shown="真" w219 {
          tunnel: w217 -> [_ w235]
          frame False {
          }
          frame True {
            n300 = flat-sequence {
              tunnel: w235 -> [w236]
              frame #0 {
                n301 = call "CODMn电源命令.vi"("通电/断电"=TRUE, "队列"=w236) -> ()  [unwired: 9 in, 1 out]
              }
              frame #1 {
                n302 = Wait (ms)(milliseconds to wait=u32 90000 ("等待时间（毫秒）")) -> ()  [unwired: 1 out]
              }
              frame #2 {
                n303 = global read "COD浓度全局变量.vi" "COD浓度（mg/L)"() -> (w240:dbl)
                n304 = Greater Or Equal?(x=w240, y=10.0) -> (x >= y?=w242:bool)
                n305 = case shown="假" w242 {
                  tunnel: [enum32{"H", "L", "AUTO"}."L" ("CODMn量程切换") enum32{"H", "L", "AUTO"}."H" ("CODMn量程切换")] -> w239
                  frame False {
                  }
                  frame True {
                  }
                }
                n306 = call "CODMn启动命令 (子VI).vi"("CODMn量程切换"=w239, "启动测量模式"=T10 {"测量模式"=enum."跨度核查"}) -> ()  [unwired: 10 in]
              }
            }
          }
        }
      }
    }
    n307 = case shown="真" w188 {
      tunnel: w186 -> [_ w282]
      tunnel: w185 -> [_ w281]
      tunnel: w170 -> [_ w279]
      tunnel: w169 -> [_ w278]
      frame False {
      }
      frame True {
        n308 = local read "总氮"() -> (w280:bool)
        n309 = local read "氨氮"() -> (w286:bool)
        n310 = local read "总磷"() -> (w285:bool)
        n311 = local read "CODmn"() -> (w284:bool)
        n312 = local read "CODCr"() -> (w283:bool)
        n313 = case shown="真" w280 {
          tunnel: w278 -> [_ w287]
          frame False {
          }
          frame True {
            n314 = flat-sequence {
              tunnel: w287 -> [w293]
              frame #0 {
                n315 = Wait (ms)(milliseconds to wait=u32 30000 ("等待时间（毫秒）")) -> ()  [unwired: 1 out]
              }
              frame #1 {
                n316 = global read "系统设置全局变量.vi" "总氮自动测试量程配置"() -> (w292:T13)
                n317 = Unbundle By Name(w292) -> ("空白核查量程模式"=w289:enum16{"H", "L", "AUTO"})
                n318 = Bundle By Name(cluster=T9 {"站号"=2, "量程切换"=enum."L", "控制命令"=enum."空白测试", "模式设置"=enum."待机", "测量间隔"=0} ("参数"), "量程切换"=w289) -> (w290:T9)
                n319 = call "总氮启动命令.vi"("参数"=w290) -> ("启动命令"=w294:cluster{"命令":string, "data":variant})  [unwired: 10 in]
                n320 = Enqueue Element(queue=w293, element=w294) -> ()  [unwired: 2 in, 3 out]
              }
            }
          }
        }
        n321 = case shown="真" w286 {
          tunnel: w282 -> [_ w328]
          tunnel: w281 -> [_ w327]
          frame False {
          }
          frame True {
            n322 = flat-sequence {
              tunnel: w328 -> [w329]
              tunnel: w327 -> [w336]
              frame #0 {
                n323 = call "氨氮电源命令.vi"("通电/断电"=TRUE, "队列"=w329) -> ()  [unwired: 9 in, 1 out]
              }
              frame #1 {
                n324 = Wait (ms)(milliseconds to wait=u32 30000 ("等待时间（毫秒）")) -> ()  [unwired: 1 out]
              }
              frame #2 {
                n325 = global read "系统设置全局变量.vi" "氨氮自动测试量程配置"() -> (w335:T13)
                n326 = Unbundle By Name(w335) -> ("空白核查量程模式"=w333:enum16{"H", "L", "AUTO"})
                n327 = Bundle By Name(cluster=T9 {"站号"=3, "量程切换"=enum."L", "控制命令"=enum."空白测试", "模式设置"=enum."受控模式", "测量间隔"=0} ("参数"), "量程切换"=w333) -> (w332:T9)
                n328 = call "总磷氨氮启动命令.vi"("参数"=w332) -> ("启动命令"=w337:cluster{"命令":string, "data":variant})  [unwired: 10 in]
                n329 = Enqueue Element(queue=w336, element=w337) -> ()  [unwired: 2 in, 3 out]
              }
            }
          }
        }
        n330 = case shown="真" w285 {
          tunnel: w282 -> [_ w307]
          tunnel: w279 -> [_ w306]
          frame False {
          }
          frame True {
            n331 = flat-sequence {
              tunnel: w307 -> [w309]
              tunnel: w306 -> [w311]
              frame #0 {
                n332 = call "总磷总氮电源命令.vi"("通电/断电"=TRUE, "队列"=w309) -> ()  [unwired: 9 in, 1 out]
              }
              frame #1 {
                n333 = Wait (ms)(milliseconds to wait=u32 30000 ("等待时间（毫秒）")) -> ()  [unwired: 1 out]
              }
              frame #2 {
                n334 = disable-structure shown="启用" {
                  disable-tunnel: w311 -> [_ w325]
                  frame Disabled {
                    n335 = vi-ref "斯坦道仪器.lvlib:总磷氨氮测量流程.vi"() -> (w316:refnum<vi>)
                    n336 = property class="VI"(reference=w316) -> ("Name"=w317:string)  [unwired: 1 in, 2 out]
                    n337 = Open VI Reference(type specifier VI Refnum (for type only)=refnum<vi> refnum ("类型说明符VI引用句柄（仅用于类型）"), vi path=w317, options=128 ("选项")) -> (vi reference=w314:refnum<vi>)  [unwired: 3 in, 1 out]
                    n338 = call-by-ref "开始异步调用"(reference=w314, "量程模式"=T11 {"水样测试量程切换模式"=enum."AUTO", "空白核查量程切换模式"=enum."L", "跨度核查量程切换模式"=enum."H"}, "参数"=T9 {"站号"=2, "量程切换"=enum."L", "控制命令"=enum."零点核查", "模式设置"=enum."受控模式", "测量间隔"=0}) -> (reference out=w313:refnum<vi>, error out=w312:errorcluster)  [unwired: 11 in]
                    n339 = Close Reference(reference=w313, error in (no error)=w312) -> ()  [unwired: 1 out]
                  }
                  frame Enabled {
                    n340 = global read "系统设置全局变量.vi" "总磷自动测试量程配置"() -> (w324:T13)
                    n341 = Unbundle By Name(w324) -> ("空白核查量程模式"=w323:enum16{"H", "L", "AUTO"})
                    n342 = Bundle By Name(cluster=T9 {"站号"=1, "量程切换"=enum."L", "控制命令"=enum."空白测试", "模式设置"=enum."待机", "测量间隔"=0} ("参数"), "站号"=w323) -> (w321:T9)
                    n343 = call "总磷氨氮启动命令.vi"("参数"=w321) -> ("启动命令"=w326:cluster{"命令":string, "data":variant})  [unwired: 10 in]
                    n344 = Enqueue Element(queue=w325, element=w326) -> ()  [unwired: 2 in, 3 out]
                  }
                }
              }
            }
          }
        }
        n345 = case shown="真" w284 {
          tunnel: w282 -> [_ w300]
          frame False {
          }
          frame True {
            n346 = flat-sequence {
              tunnel: w300 -> [w301]
              frame #0 {
                n347 = call "CODMn电源命令.vi"("通电/断电"=TRUE, "队列"=w301) -> ()  [unwired: 9 in, 1 out]
              }
              frame #1 {
                n348 = Wait (ms)(milliseconds to wait=u32 90000 ("等待时间（毫秒）")) -> ()  [unwired: 1 out]
              }
              frame #2 {
                n349 = call "CODMn启动命令 (子VI).vi"("CODMn量程切换"=enum32{"H", "L", "AUTO"}."L", "启动测量模式"=T10 {"测量模式"=enum."空白测试"}) -> ()  [unwired: 10 in]
              }
            }
          }
        }
        n350 = case shown="真" w283 {
          tunnel: w282 -> [_ w295]
          frame False {
          }
          frame True {
            n351 = flat-sequence {
              tunnel: w295 -> [w296]
              frame #0 {
                n352 = call "CODCr电源命令.vi"("通电/断电"=TRUE, "队列"=w296) -> ()  [unwired: 9 in, 1 out]
              }
              frame #1 {
                n353 = Wait (ms)(milliseconds to wait=u32 90000 ("等待时间（毫秒）")) -> ()  [unwired: 1 out]
              }
              frame #2 {
                n354 = call "CODCr启动命令 (子VI).vi"("启动测量模式"=T10 {"测量模式"=enum."空白测试"}) -> ()  [unwired: 11 in]
              }
            }
          }
        }
      }
    }
    n355 = case shown="真" w191 {
      tunnel: w194 -> [_ w339]
      tunnel: w186 -> [_ w338]
      frame False {
      }
      frame True {
        n356 = flat-sequence {
          tunnel: w339 -> [w346]
          tunnel: w338 -> [w340]
          frame #0 {
            n357 = Cancel Notification(0:w346) -> ()  [unwired: 1 in, 3 out]
            n358 = call "CODMn电源命令.vi"("通电/断电"=TRUE, "队列"=w340) -> ()  [unwired: 9 in, 1 out]
            n359 = call "氨氮电源命令.vi"("通电/断电"=TRUE, "队列"=w340) -> ()  [unwired: 9 in, 1 out]
            n360 = call "总磷总氮电源命令.vi"("通电/断电"=TRUE, "队列"=w340) -> ()  [unwired: 9 in, 1 out]
            n361 = call "多参数电源命令.vi"("通电/断电"=TRUE, "队列"=w340) -> ()  [unwired: 9 in, 1 out]
            n362 = call "CODCr电源命令.vi"("通电/断电"=TRUE, "队列"=w340) -> ()  [unwired: 9 in, 1 out]
          }
          frame #1 {
            n363 = vi-ref "PLC.lvlib:一体站流程自动启动.vi"() -> (w356:refnum<vi>)
            n364 = property class="VI"(reference=w356) -> ("Name"=w357:string)  [unwired: 1 in, 2 out]
            n365 = Bundle By Name(cluster=T12 {"CODCr"={"启动测量模式"={"测量模式"=enum."水样测量"}, "确定按钮"=FALSE}, "参数启用"={"多参数"=FALSE, "CODMn"=FALSE, "总磷"=FALSE, "总氮"=FALSE, "氨氮"=FALSE, "CODcr"=FALSE}} ("参数"), "CODCr.启动测量模式"=T10 {"测量模式"=enum."水样测量"}, "参数启用.多参数"="多参数", "参数启用.CODMn"="CODmn", "参数启用.总磷"="总磷", "参数启用.氨氮"="氨氮", "参数启用.CODcr"="CODCr", "参数启用.总氮"="总氮") -> (w348:T12)
            n366 = Open VI Reference(type specifier VI Refnum (for type only)=refnum<vi> refnum ("类型说明符VI引用句柄（仅用于类型）"), vi path=w357, options=128 ("选项")) -> (vi reference=w354:refnum<vi>, error out=w353:errorcluster)  [unwired: 3 in]
            n367 = call-by-ref "开始异步调用"(reference=w354, error in=w353, "参数"=w348) -> (reference out=w352:refnum<vi>, error out=w351:errorcluster)  [unwired: 11 in]
            n368 = Close Reference(reference=w352, error in (no error)=w351) -> ()  [unwired: 1 out]
          }
        }
      }
    }
  }
